vi "configTabUI.vi"(11 "ConfigurationTabUI in":refnum<class "ConfigurationTabUI.lvclass">) -> ()   [LabVIEW 2015, in "ExampleConfiguration.lvlib" / "ConfigurationTabUI.lvclass"]
doc: "Presents the configuration information for the current component to the user."
uses:
  ConfigurationTabUI.lvclass
  ComponentTemplateCore/ComponentModel/ComponentModelRT/ComponentConfigurationTypedefs/IRQConfig.ctl
  ComponentTemplateCore/ComponentModel/ComponentModelRT/ComponentConfigurationTypedefs/LoopConfig.ctl
  ComponentTemplateCore/ComponentModel/ComponentModelRT/ComponentConfigurationTypedefs/RIOConfig.ctl
  ComponentTemplateCore/ComponentModel/ComponentModel/Typedefs/CommunicationConfig.ctl
  ComponentTemplateCore/ComponentModel/ComponentModel/Typedefs/HeartbeatConfig.ctl
  ComponentTemplateCore/ConfigurationWithXML/MyComputer/Configuration/ConfigurationTabUI/ConfigurationTabUI.lvclass
panel:
  out "error out":errorcluster
  out "cfgDataTabControl":T1(tab)
  in  "communicationConfig":T2 {"InstanceIdentifier" min=-1}
  in  "heartbeatConfig":T3={"Heartbeat Interval (s)"=1.0, "Heartbeat Timeout (s)"=5.0} {"Heartbeat Timeout (s)" min=0.5 max=60.0 step=0.1 format="%.1f"; "Heartbeat Interval (s)" min=0.1 max=10.0 step=0.1 format="%.1f"}
  in  "irqConfig":T4={"irqNumber"=0, "irqTimeout_ms"=1000} {"irqTimeout_ms" min=-1; "irqNumber" min=0 max=31}
  in  "loopConfig":T5={"hostLoopPeriod_s"=0.016, "hostLoopPeriodAllowedJitter_percent"=10.0} {"hostLoopPeriodAllowedJitter_percent" min=1.0 max=100.0; "hostLoopPeriod_s" min=0.001 max=600.0}
  in  "rioConfig":T6={"rioResourceName"="RIO0"}
  in  "EditWarningsConfig":bool
  in  "warningsDisplayConfig":refnum<k21>[](array[refnum])
  # "(-1 for none)"
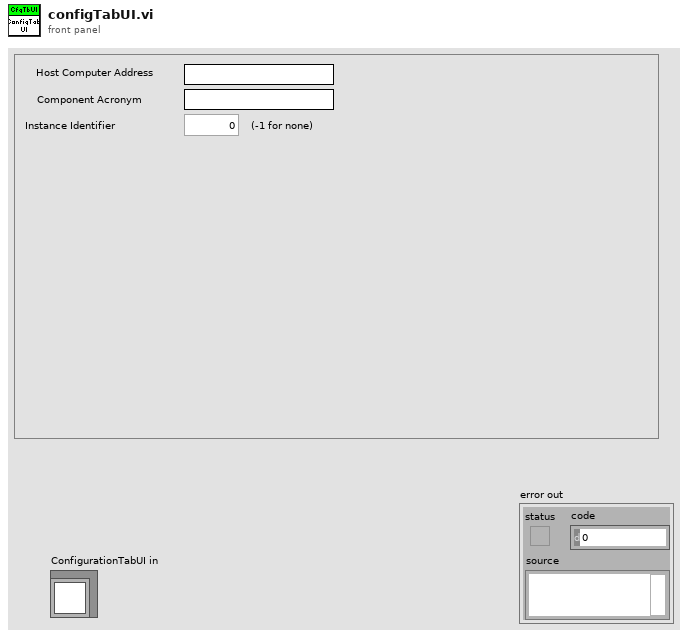
[diagram p1: front panel]
types:
  T1 = enum32{"Communication", "Heartbeat", "IRQ", "Loop", "RIO", "Warnings Display"}
  T2 = typedef "CommunicationConfig.ctl" = cluster{"hostComputerAddress":string, "ComponentAcronym":string, "InstanceIdentifier":i32}
  T3 = typedef "heartbeatConfig.ctl" = cluster{"Heartbeat Interval (s)":dbl, "Heartbeat Timeout (s)":dbl}
  T4 = typedef "irqConfig.ctl" = cluster{"irqNumber":i32, "irqTimeout_ms":i32}
  T5 = typedef "LoopConfig.ctl" = cluster{"hostLoopPeriod_s":dbl, "hostLoopPeriodAllowedJitter_percent":dbl}
  T6 = typedef "rioConfig.ctl" = cluster{"rioResourceName":string}
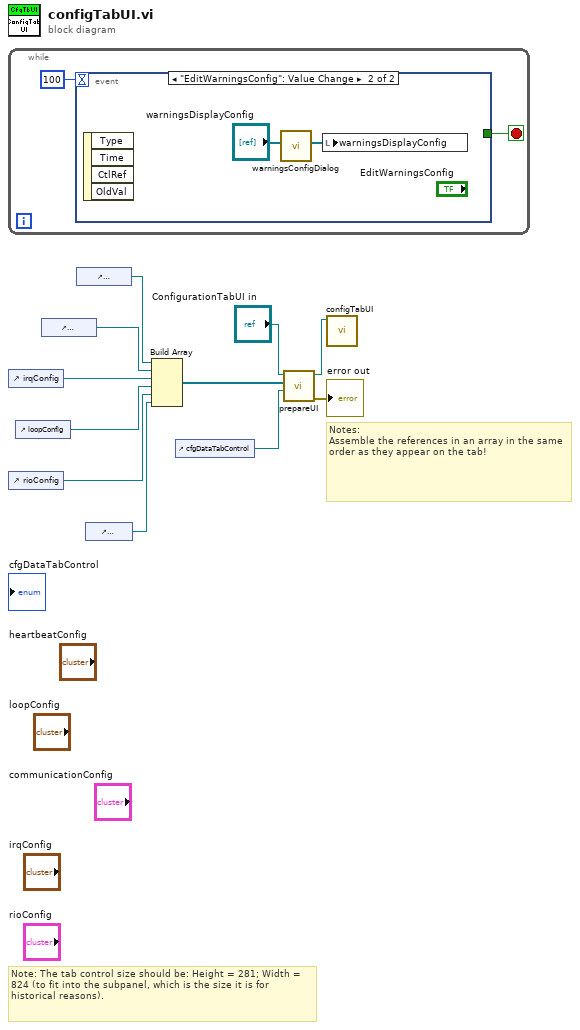
[diagram p0: block diagram]
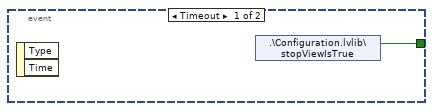
[diagram p2: hidden frame]
diagram:
  # "Note: The tab control size should be: Height = 281; Width = 824 (to fit into the subpanel, which is the size it is for historical reasons)."
  # "Notes:\nAssemble the references in an array in the same order as they appear on the tab!"
  n1 = while {
    stop <- w12 stop-if-true
    n2 = event shown="[1] \"EditWarningsConfig\": Value Change" {
      selector: _ -> [_ _]
      dyn-events: _ -> [_ _]
      timeout: 100 -> [_ _]
      tunnel: [w14 _] -> w12
      event Timeout {
        n3 = event-data() -> ()  [unwired: 1 in, 2 out]
        n4 = shared-variable ".\\Configuration.lvlib\\stopViewIsTrue"() -> (w14:bool)  [unwired: 1 in, 1 out]
      }
      event "EditWarningsConfig": Value Change {
        n5 = event-data() -> ()  [unwired: 1 in, 4 out]
        n6 = call "warningsConfigDialog.vi"("data"="warningsDisplayConfig") -> ("data out"=w15:refnum<k21>[])  [unwired: 10 in]
        n7 = local write "warningsDisplayConfig"(w15) -> ()
      }
    }
  }
  n8 = control-ref of="irqConfig"() -> (w6:refnum<vi>)
  n9 = control-ref of="rioConfig"() -> (w4:refnum<vi>)
  n10 = control-ref of="loopConfig"() -> (w5:refnum<vi>)
  n11 = control-ref of="heartbeatConfig"() -> (w7:refnum<vi>)
  n12 = control-ref of="communicationConfig"() -> (w8:refnum<vi>)
  n13 = control-ref of="warningsDisplayConfig"() -> (w3:refnum<vi>)
  n14 = Build Array(w8, w7, w6, w5, w4, w3) -> (w9:refnum<vi>[])
  n15 = control-ref of="cfgDataTabControl"() -> (w11:refnum<vi>)
  n16 = call "prepareUI.vi"("tabCtlRefnum"=w11, "controlRef"=w9, "ConfigurationTabUI in"="ConfigurationTabUI in") -> ("error out"=→"error out":errorcluster, "ConfigurationTabUI out"=w1:refnum<class "ConfigurationTabUI.lvclass">)  [unwired: 7 in]
  n17 = call-parent "configTabUI.vi"("ConfigurationTabUI in"=w1) -> ()  [unwired: 11 in]
